vi "uActor_Def_uErr.vi"(8 "error in (no error)":errorcluster, 11 "uActor in":refnum<class "uActor.lvclass">) -> (0 "error out":errorcluster, 3 "uActor out":refnum<class "uActor.lvclass">)   [LabVIEW 2023, in "uLib.lvlib" / "uActor.lvclass"]
doc: "Dynamic dispatch method to allow children actors to forcefully associate to themselves an Error handling behavior by writing a uErr child to themselves prior to the prelaunch init.\n\nA child actor may decide to be more lenient and force its predefined Err handling behavior only if no behavior has been specified at runtime before launching the actor.\n\nNote that a nested actor by default gets assigned the runtime error behavior of its caller actor prior to getting launched."
uses:
  uActor.lvclass
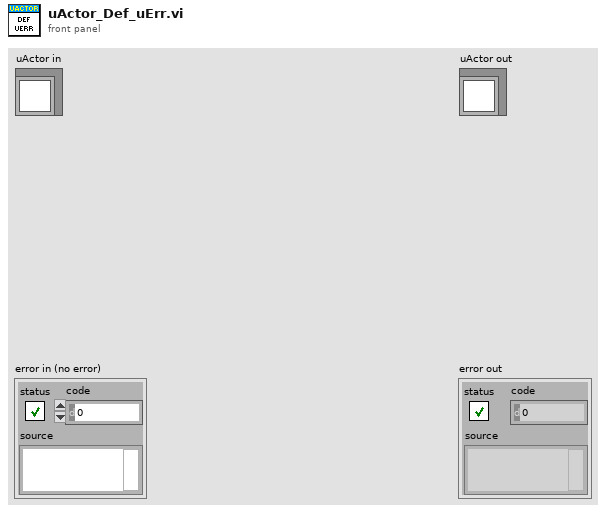
[diagram p1: front panel]
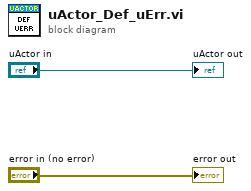
[diagram p0: block diagram]
diagram:
  "error out" <- "error in (no error)"
  "uActor out" <- "uActor in"
